vi "TDMS_writeWave.vi"() -> ()   [LabVIEW 2011]
panel:
  out "error out":errorcluster
  in  "stop":bool
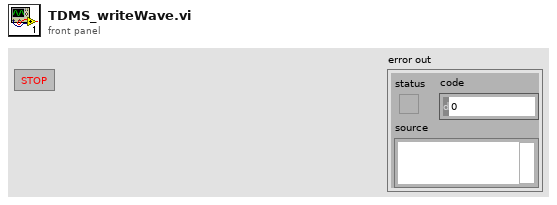
[diagram p1: front panel]
types:
  T1 = enum16{"open", "open or create", "create or replace", "create", "open (read-only)"}
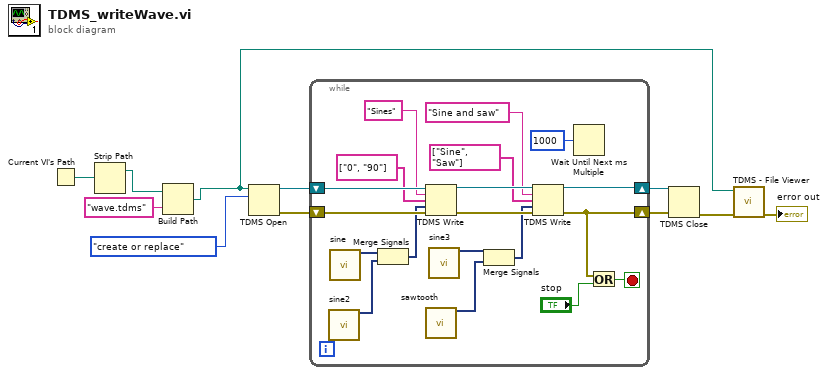
[diagram p0: block diagram]
diagram:
  n1 = Current VI's Path() -> (path=w11:path)
  n2 = Strip Path(path=w11) -> (stripped path=w10:path)  [unwired: 1 out]
  n3 = Build Path(base path=w10, name or relative path="wave.tdms") -> (appended path=w3:path)
  n4 = TDMS Open(10:T1."create or replace" ("operation (0:open)"), 11:w3) -> (0:w6:errorcluster, 3:w7:refnum<k34>)  [unwired: 4 in]
  n5 = while {
    shift-right: [w25] -> w4
    shift-left: w7 -> [w30]
    shift-right: [w14] -> w5
    shift-left: w6 -> [w29]
    stop <- w12 stop-if-true
    n6 = call "sine2"() -> ("Sine"=w24:dynamicdata)  [unwired: 14 in, 1 out]
    n7 = call "sine"() -> ("Sine"=w23:dynamicdata)  [unwired: 14 in, 1 out]
    n8 = Merge Signals(w23, w24) -> (w22:dynamicdata)
    n9 = TDMS Write(0:w30, 5:"Sines" ("group name in (Untitled)"), 7:string[] ["0", "90"] ("channel name(s) in (Untitled)"), 9:w22, 11:w29) -> (4:w28:refnum<k34>, 15:w27:errorcluster)  [unwired: 1 in, 2 out]
    n10 = call "sawtooth"() -> ("Sawtooth"=w19:dynamicdata)  [unwired: 14 in, 1 out]
    n11 = call "sine3"() -> ("Signal"=w20:dynamicdata)  [unwired: 14 in, 1 out]
    n12 = Merge Signals(w20, w19) -> (w18:dynamicdata)
    n13 = TDMS Write(0:w28, 5:"Sine and saw" ("group name in (Untitled)"), 7:string[] ["Sine", "Saw"] ("channel name(s) in (Untitled)"), 9:w18, 11:w27) -> (4:w25:refnum<k34>, 15:w14:errorcluster)  [unwired: 1 in, 2 out]
    n14 = Wait Until Next ms Multiple(millisecond multiple=u32 1000) -> ()  [unwired: 1 out]
    n15 = Or(x=w14, y="stop") -> (x .or. y?=w12:bool)
  }
  n16 = TDMS Close(8:w5, 11:w4) -> (0:w2:errorcluster)  [unwired: 1 out]
  n17 = call <vilib>:"TDMS - File Viewer.vi"("error in (no error)"=w2, "file path"=w3) -> ("error out"=→"error out":errorcluster)  [unwired: 4 in, 1 out]
